vi "Set One Filter.vi"(8 "error in (no error)":errorcluster, 9 "Position (0:4)":i32, 10 "Filter Wheel (0:n-1)":i32, 11 "Filter Wheel Simulator in":refnum<class "Filter Wheel Simulator.lvclass">) -> (0 "error out":errorcluster, 1 "Target Counts":i32, 2 "Curr Pos":i32, 3 "Filter Wheel Simulator out":refnum<class "Filter Wheel Simulator.lvclass">, 4 "Message":string, 6 "No Move?":bool)   [LabVIEW 2024, in "Filter Wheel Simulator.lvclass"]
uses:
  Filter Wheel Simulator.lvclass
  Filter Wheel Simulator.lvclass/Filter Wheel Simulator.ctl
  Filter Wheel Object/Filter Wheel.lvclass
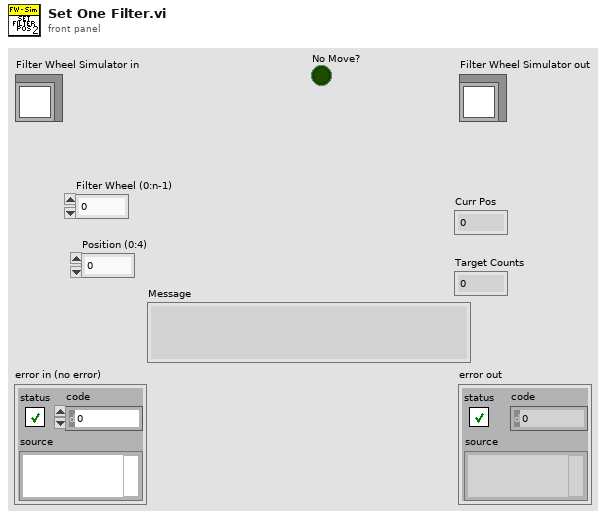
[diagram p1: front panel]
types:
  T1 = typedef "Filter Wheel Simulator.lvclass/Filter Wheel cluster Simulated Status.ctl" = cluster{"Move Start Time":timestamp, "Moving?":bool, "Target Pos":dbl, "Direction":bool}
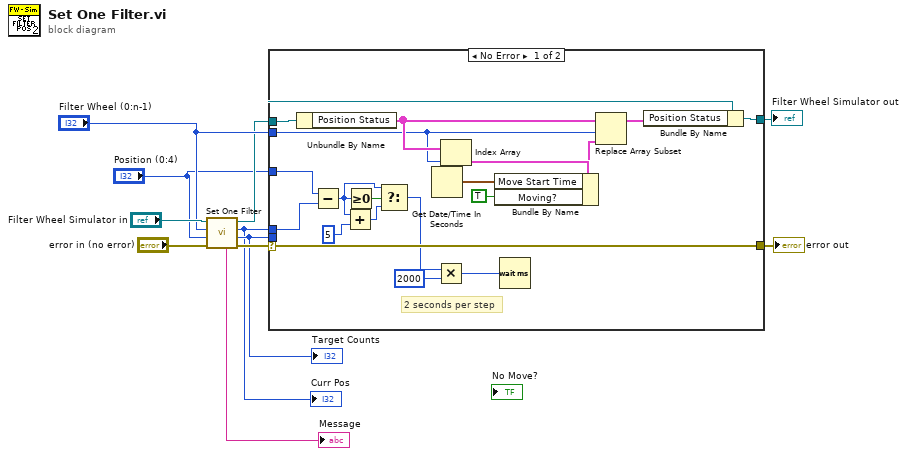
[diagram p0: block diagram]
diagram:
  n1 = call-parent "Set One Filter.vi"("error in (no error)"="error in (no error)", "Position (0:4)"="Position (0:4)", "Filter Wheel (0:n-1)"="Filter Wheel (0:n-1)", "Filter Wheel in"="Filter Wheel Simulator in") -> ("error out"=w6:errorcluster, "Target Counts"=w4:i32, "Curr Pos"=w3:i32, "Filter Wheel out"=w8:refnum<class "Filter Wheel Simulator.lvclass">, "Message"=→"Message":string)  [unwired: 2 in, 1 out]
  "Target Counts" <- w4
  "Curr Pos" <- w3
  n2 = case shown="No Error" w6 {
    selector: w6 -> [w21 w32]
    tunnel: w4 -> [_ _]
    tunnel: "Filter Wheel (0:n-1)" -> [w26 _]
    tunnel: w8 -> [w24 w31]
    tunnel: [w22 w31] -> w7
    tunnel: [w21 w32] -> w5
    tunnel: w3 -> [w19 _]
    tunnel: "Position (0:4)" -> [w20 _]
    frame No Error {
      # "2 seconds per step"
      n3 = Unbundle By Name(w24) -> ("Position Status"=w27:T1[])
      n4 = Subtract(x=w20, y=w19) -> (x-y=w15:i32)
      n5 = Add(x=w15, y=5) -> (x+y=w16:i32)
      n6 = Greater Or Equal To 0?(x=w15) -> (x >= 0?=w17:bool)
      n7 = Select(t=w15, s=w17, f=w16) -> (s? t:f=w14:i32)
      n8 = Get Date/Time In Seconds() -> (seconds since 1Jan1904=w30:timestamp)
      n9 = Multiply(x=w14, y=2000) -> (x*y=w12:i32)
      n10 = Index Array(array=w27, index=w26) -> (element=w28:T1)
      n11 = Bundle By Name(cluster=w28, "Move Start Time"=w30, "Moving?"=TRUE) -> (w25:T1)
      n12 = Wait (ms)(milliseconds to wait=w12) -> ()  [unwired: 1 out]
      n13 = Replace Array Subset(array=w27, new element=w25, index=w26) -> (w23:T1[])
      n14 = Bundle By Name(cluster=w24, "Position Status"=w23) -> (w22:refnum<class "Filter Wheel Simulator.lvclass">)
    }
    frame Error {
    }
  }
  "error out" <- w5
  "Filter Wheel Simulator out" <- w7
